vi "Convert CFA to U32.vi"(2 "CFA in":T1 {"CFA" items=["CFA_NONE", "CFA_VRI", "CFA_VRIV6", "CFA_BAYER", "CFA_BAYERFLIP"]}) -> (16 "CFA out":u32 format="%x")   [LabVIEW 2013, in "VRI.lvlib"]
uses:
  VRI.lvlib
  _Type Defs/PhInt CFA.ctl
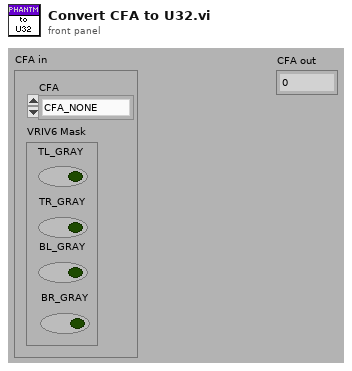
[diagram p1: front panel]
types:
  T1 = typedef "VRI.lvlib/PhInt CFA.ctl" = cluster{"CFA":u32, "VRIV6 Mask":cluster{"TL_GRAY":bool, "TR_GRAY":bool, "BL_GRAY":bool, "BR_GRAY":bool}}
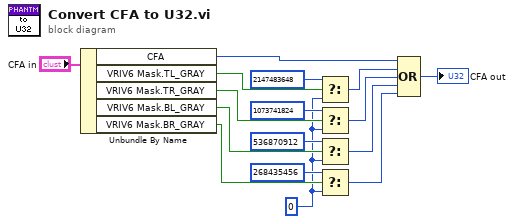
[diagram p0: block diagram]
diagram:
  w1 = u32 0 ("f")
  n1 = Unbundle By Name("CFA in") -> ("CFA"=w7:u32, "VRIV6 Mask.TL_GRAY"=w15:bool, "VRIV6 Mask.TR_GRAY"=w12:bool, "VRIV6 Mask.BL_GRAY"=w13:bool, "VRIV6 Mask.BR_GRAY"=w14:bool)
  n2 = Select(t=u32 2147483648, s=w15, f=w1) -> (s? t:f=w6:u32)
  n3 = Select(t=u32 1073741824, s=w12, f=w1) -> (s? t:f=w5:u32)
  n4 = Select(t=u32 536870912, s=w13, f=w1) -> (s? t:f=w4:u32)
  n5 = Select(t=u32 268435456, s=w14, f=w1) -> (s? t:f=w3:u32)
  n6 = Compound Arithmetic op=OR(w7, w6, w5, w4, w3) -> (→"CFA out":u32)
